vi "acquireValue.vi"(8 "error in (no error)":errorcluster, 10 "nextSample?":bool, 11 "heartbeat in":refnum<class "heartbeat.lvclass">) -> (0 "error out":errorcluster, 1 "function return":i32, 2 "variantData":variant, 3 "heartbeat out":refnum<class "heartbeat.lvclass">)   [LabVIEW 2016, in "SALLV_MtAtElectrometer_Messaging.lvlib" / "heartbeat.lvclass"]
uses:
  heartbeat.lvclass
  heartbeat.lvclass/heartbeat.ctl
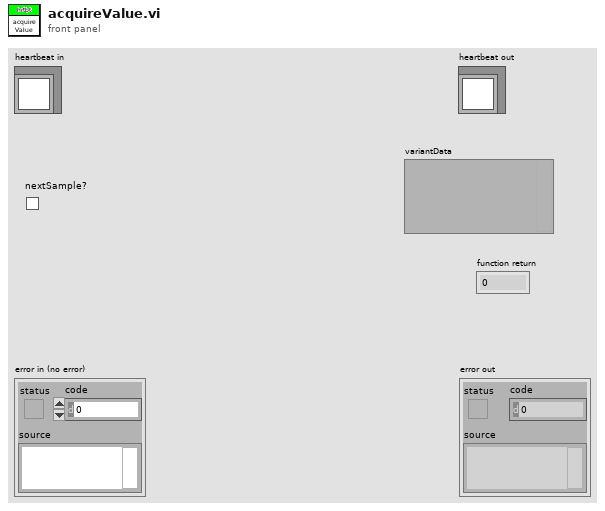
[diagram p1: front panel]
types:
  T1 = typedef "SALLV_EXA.lvlib/logevent_heartbeat.ctl" = cluster{"heartbeat":bool, "priority":i32}
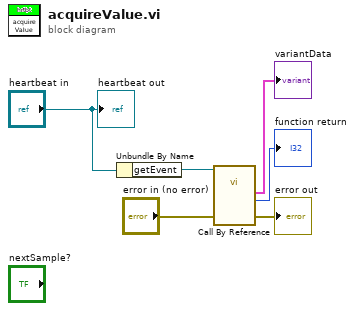
[diagram p0: block diagram]
diagram:
  n1 = Unbundle By Name("heartbeat in") -> ("getEvent"=w6:refnum<vi>)
  n2 = call-by-ref "?"(reference=w6, "error in (no error)"="error in (no error)") -> ("error out"=→"error out":errorcluster, "function return"=→"function return":i32, "logevent_heartbeat_Ctl out"=→"variantData":T1)  [unwired: 9 in, 2 out]
  "heartbeat out" <- "heartbeat in"
